vi "Get Diff Report.vi"(8 "error in (no error)":errorcluster, 10 "RSL Path":path, 11 "Ref RSL Path":path) -> (0 "error out":errorcluster)   [LabVIEW 2019]
uses:
  <vilib>/addons/analyzer/NI_VIAnalyzerTKVIs.lvlib
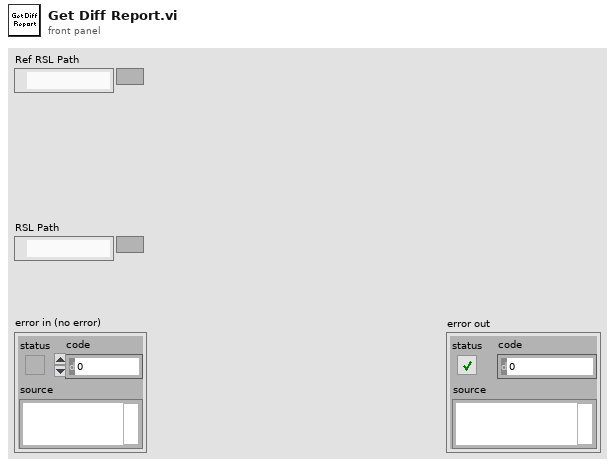
[diagram p1: front panel]
types:
  T1 = typedef "VIAnCtl Results.ctl" = cluster{"Test Name":string, "Results Data":T2[], "Status":T3, "Exceed Max Fails?":bool}
  T2 = typedef "VIAnCtl ResultsData (index).ctl" = cluster{"Result Message":string, "Ref Index":i32}
  T3 = typedef "VIAnCtl ResultStatus.ctl" = enum16{"Pass", "Fail", "Skipped", "VI not loadable", "Test not loadable", "Test not runnable", "Test error out"}
  T4 = typedef "VIAnRes Parsed Results Data (by VI).ctl" = cluster{"VI Path":path, "Pass":cluster{"row":i32, "column":i32}[], "Fail":cluster{"row":i32, "column":i32}[], "Skipped":cluster{"row":i32, "column":i32}[], "VI not loadable":cluster{"row":i32, "column":i32}[], "Test not loadable":cluster{"row":i32, "column":i32}[], "Test not runnable":cluster{"row":i32, "column":i32}[], "Test error out":cluster{"row":i32, "column":i32}[]}
  T5 = typedef "VIAnRes Parsed Results Data (by Test).ctl" = cluster{"Test Name":string, "Pass":cluster{"VI Path":path, "index":cluster{"row":i32, "column":i32}}[], "Fail":cluster{"VI Path":path, "index":cluster{"row":i32, "column":i32}}[], "Skipped":cluster{"VI Path":path, "index":cluster{"row":i32, "column":i32}}[]}
  T6 = typedef "VIAnCtl Test Config Data.ctl" = cluster{"Test Name":string, "Config Ref":refnum<vi>, "Ref Valid?":bool, "Test Ranking":T7, "Max Failures":u32, "Test Path":path, "Control Values":T8[], "Selected?":bool}
  T7 = typedef "VIAnCtl TestRanking.ctl" = u16
  T8 = typedef "VIAnCtl Config Control Value.ctl" = cluster{"Control Name":string, "Control Value":variant}
  T9 = cluster{"Raw Results":T1[][], "Parsed Results Data (by VI)":T4[], "Parsed Results Data (by Test)":T5[], "Summary Statistics":cluster{"Passed Tests":i32, "Failed Tests":i32, "Skipped Tests":i32, "VIs not loadable":i32, "Tests not loadable":i32, "Tests not runnable":i32, "Test error out":i32, "Start Time":u32, "Total Time (s)":dbl}, "Test Config Data":T6[]}
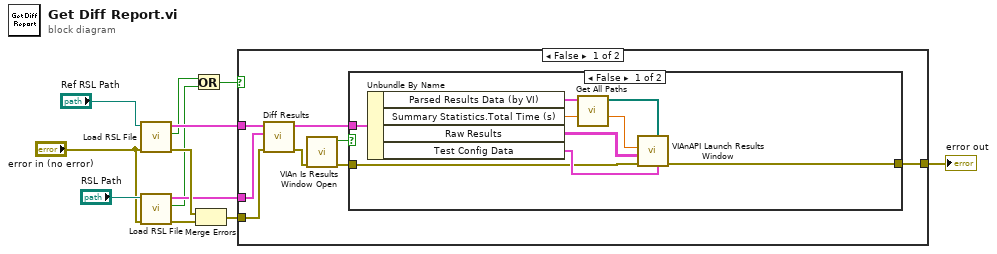
[diagram p0: block diagram]
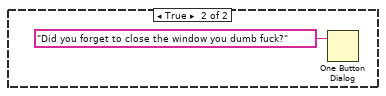
[diagram p2: hidden frame]
diagram:
  n1 = call "Load RSL File.vi"("error in (no error)"="error in (no error)", "RSL Path"="Ref RSL Path") -> ("error out"=w11:errorcluster, "invalid file?"=w7:bool, "RSL Data"=w10:T9)  [unwired: 7 in]
  n2 = call "Load RSL File.vi"("error in (no error)"="error in (no error)", "RSL Path"="RSL Path") -> ("error out"=w3:errorcluster, "invalid file?"=w5:bool, "RSL Data"=w8:T9)  [unwired: 7 in]
  n3 = Or(x=w7, y=w5) -> (x .or. y?=w6:bool)
  n4 = Merge Errors(w11, w3) -> (w4:errorcluster)
  n5 = case shown="False" w6 {
    tunnel: w4 -> [w18 w30]
    tunnel: w10 -> [w17 _]
    tunnel: w8 -> [w16 _]
    tunnel: [w13 w30] -> w1
    frame False {
      n6 = call "Diff Results.vi"("error in (no error)"=w18, "RSL Data in"=w16, "Reference RSL Data in"=w17) -> ("error out"=w14:errorcluster, "RSL Data out"=w15:T9)  [unwired: 7 in]
      n7 = call <vilib>:"VIAn Is Results Window Open.vi"("error in (no error)"=w14) -> ("error out"=w20:errorcluster, "VI Analyzer Results Window open?"=w19:bool)  [unwired: 9 in]
      n8 = case shown="False" w19 {
        tunnel: w15 -> [w25 _]
        tunnel: w20 -> [w24 _]
        tunnel: [w21 _] -> w13
        frame False {
          n9 = Unbundle By Name(w25) -> ("Parsed Results Data (by VI)"=w23:T4[], "Summary Statistics.Total Time (s)"=w27:dbl, "Raw Results"=w28:T1[][], "Test Config Data"=w26:T6[])
          n10 = call "Get All Paths.vi"("Parsed Results Data (by VI)"=w23) -> ("Array"=w22:path[])  [unwired: 10 in]
          n11 = call <vilib>:"VIAnAPI Launch Results Window.vi"("API Test Config Data"=w26, "VIs Tested"=w22, "error in (no error)"=w24, "Results Array"=w28, "Total Time"=w27) -> ("error out"=w21:errorcluster)  [unwired: 6 in]
        }
        frame True {
          n12 = One Button Dialog(message="Did you forget to close the window you dumb fuck?") -> ()  [unwired: 1 in, 1 out]
        }
      }
    }
    frame True {
    }
  }
  "error out" <- w1
